vi "8_二维码的识别与检测.vi"() -> ()   [LabVIEW 2020]
uses:
  <vilib>/vision/driver/NI_Vision_Acquisition_Software.lvlib
  <vilib>/vision/NI_Vision_Development_Module.lvlib
panel:
  in  "Font, Size & Style":T1={"Desired Font (Application)"=enum."Application Font", "[User-specified Font]"={"Font Name"="", "Size"=12, "Strikeout?"=FALSE, "Italic?"=FALSE, "Underline?"=FALSE, "Outline?"=FALSE, "Shadow?"=FALSE, "Bold?"=FALSE, "Rotation Angle"=0.0}, "Horizontal Alignment"=0, "Vertical Alignment"=0} {"Vertical Alignment" items=["Bottom", "Top", "Baseline"]; "Horizontal Alignment" items=["Left", "Center", "Right"]; "[User-specified Font]"."Rotation Angle" format="%.2f"}
  out "找到？":bool
  out "Data":string
  out "Image":T2(plugin-control)
  in  "停止":bool
  in  "Session In":refnum<k21>
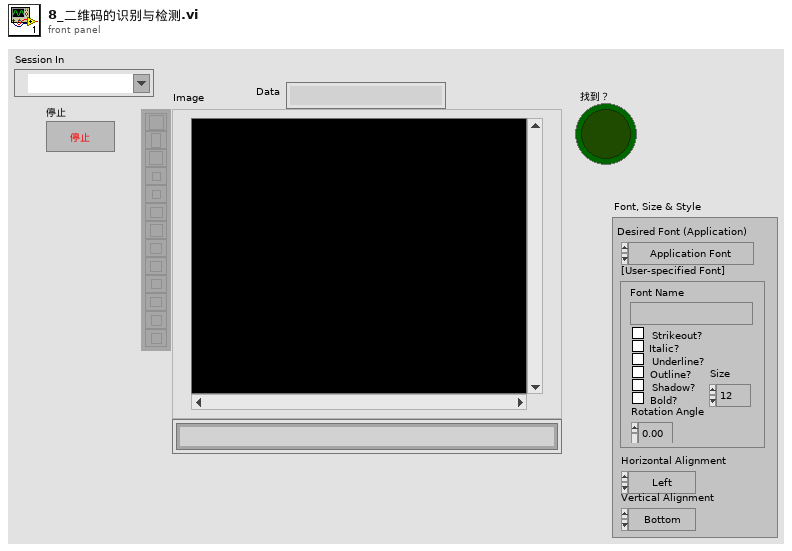
[diagram p1: front panel]
types:
  T1 = cluster{"Desired Font (Application)":enum16{"User-specified Font", "Application Font", "System Font", "Dialog Font"}, "[User-specified Font]":cluster{"Font Name":string, "Size":i16, "Strikeout?":bool, "Italic?":bool, "Underline?":bool, "Outline?":bool, "Shadow?":bool, "Bold?":bool, "Rotation Angle":dbl}, "Horizontal Alignment":i16, "Vertical Alignment":i16}
  T2 = typedef "IMAQ Image.ctl" = refnum<image>
  T3 = typedef "QR Code Report.ctl" = cluster{"Found?":bool, "Data":string, "Bounding Box":cluster{"x":sgl, "y":sgl}[], "Errors Corrected":u32, "Dimensions (Rows/Cols)":u32, "Version":u32, "QR Model":T4, "Stream Mode":T5, "Barcode Polarity":T6, "Mirrored?":bool, "Append Stream Position":u32, "Size of Append Stream":u32, "First EAN-128 ID":i32, "First Alternate Language ID":i32, "Append Stream ID":u32, "Minimum Edge Strength":u32, "Demodulation Mode":T7, "Cell Sample Size":T8, "Cell Filter Mode":T9}
  T4 = typedef "QR Code Model Type.ctl" = i32
  T5 = typedef "QR Code Stream Mode Type.ctl" = i32
  T6 = typedef "Data Matrix Polarity.ctl" = i32
  T7 = typedef "Demodulation Mode.ctl" = i32
  T8 = typedef "Cell Sample Size.ctl" = i32
  T9 = typedef "Cell Filter Mode.ctl" = i32
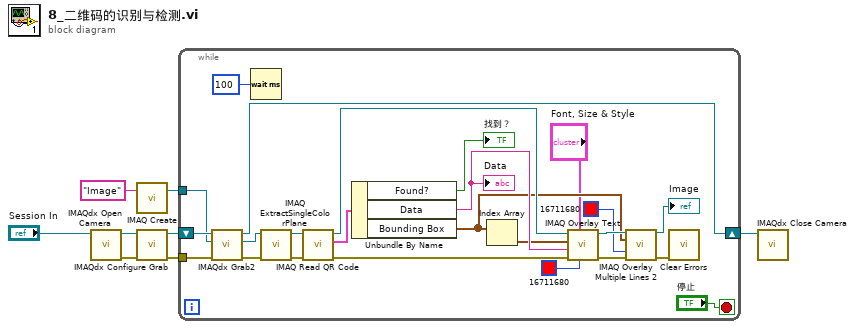
[diagram p0: block diagram]
diagram:
  n1 = call <vilib>:"IMAQdx Open Camera.vi"("Session In"="Session In") -> ("error out"=w4:errorcluster, "Session Out"=w8:refnum<k21>)  [unwired: 9 in]
  n2 = call "IMAQ Create"("Image Name"="Image") -> ("New Image"=w1:T2)  [unwired: 4 in, 1 out]
  n3 = call <vilib>:"IMAQdx Configure Grab.vi"("error in"=w4, "Session In"=w8) -> ("error out"=w5:errorcluster, "Session Out"=w7:refnum<k21>)  [unwired: 8 in]
  n4 = while {
    shift-right: [w31] -> w6
    shift-left: w7 -> [w32]
    tunnel: w5 -> [w30]
    tunnel: w1 -> [w29]
    stop <- "停止" stop-if-true
    n5 = call <vilib>:"IMAQdx Grab2.vi"("error in"=w30, "Image In"=w29, "Session In"=w32) -> ("error out"=w11:errorcluster, "Image Out"=w28:T2, "Session Out"=w31:refnum<k21>)  [unwired: 5 in, 1 out]
    n6 = Wait (ms)(milliseconds to wait=u32 100 ("等待时间（毫秒）")) -> ()  [unwired: 1 out]
    n7 = call "IMAQ ExtractSingleColorPlane"("error in (no error)"=w11, "Image Src"=w28) -> ("error out"=w12:errorcluster, "Image Dst Out"=w27:T2)  [unwired: 8 in]
    n8 = call "IMAQ Read QR Code"("error in (no error)"=w12, "Image"=w27) -> ("error out"=w10:errorcluster, "QR Code Report"=w26:T3, "Image (duplicate)"=w25:T2)  [unwired: 6 in, 1 out]
    n9 = Unbundle By Name(w26) -> ("Found?"=→"找到？":bool, "Data"=w24:string, "Bounding Box"=w19:cluster{"x":sgl, "y":sgl}[])
    "Data" <- w24
    n10 = Index Array(array=w19) -> (element=w23:cluster{"x":sgl, "y":sgl})  [unwired: 1 in]
    n11 = call "IMAQ Overlay Text"("Text Color (black)"=u32 16711680, "Font, Size & Style"="Font, Size & Style", "error in (no error)"=w10, "String"=w24, "Origin"=w23, "Image"=w25) -> ("error out"=w13:errorcluster, "Image Out"=w21:T2)  [unwired: 4 in]
    n12 = call "IMAQ Overlay Multiple Lines 2"("Image"=w21, "Line End Points"=w19, "Color"=u32 16711680, "error in (no error)"=w13) -> ("Image Out"=→"Image":T2, "error out"=w14:errorcluster)  [unwired: 10 in]
    n13 = call <vilib>:"Clear Errors.vi"("error in (no error)"=w14) -> ()  [unwired: 5 in, 2 out]
  }
  n14 = call <vilib>:"IMAQdx Close Camera.vi"("Session In"=w6) -> ()  [unwired: 10 in, 1 out]
